vi "Initialize Panel.vi"(7 "Main VI":refnum<vi>, 8 "Error In":errorcluster, 10 "Messages In":refnum<queue>, 11 "State In":T1) -> (0 "Error Out":errorcluster, 2 "Messages Out":refnum<queue>, 3 "State Out":T1)   [LabVIEW 2018, in "Bookmark Manager.lvlib"]
uses:
  Bookmark Manager.lvlib
  Controls/State.ctl
  <vilib>/addons/analyzer/_analyzerctrls.llb/VIAnCtl Analysis App Info.ctl
  Controls/Bookmark.ctl
  Controls/VI Identifier.ctl
  Controls/Bookmarks Groups.ctl
  Controls/Message.ctl
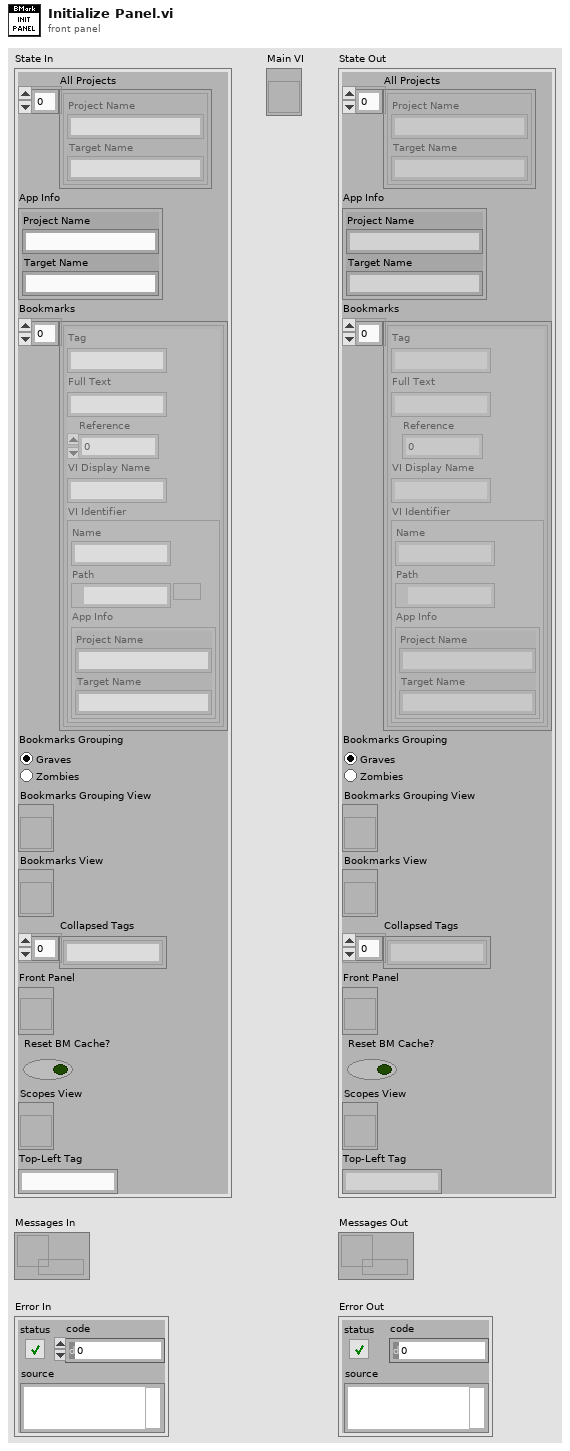
[diagram p1: front panel]
types:
  T1 = typedef "Bookmark Manager.lvlib/State.ctl" = cluster{"All Projects":T2[], "App Info":T2, "Bookmarks":T3[], "Bookmarks Grouping":T5, "Bookmarks Grouping View":refnum<vi>, "Bookmarks View":refnum<vi>, "Collapsed Tags":string[], "Front Panel":refnum<vi>, "Reset BM Cache?":bool, "Scopes View":refnum<vi>, "Top-Left Tag":string}
  T2 = typedef "VIAnCtl Analysis App Info.ctl" = cluster{"Project Name":string, "Target Name":string}
  T3 = typedef "Bookmark Manager.lvlib/Bookmark.ctl" = cluster{"Tag":string, "Full Text":string, "Reference":i32, "VI Display Name":string, "VI Identifier":T4}
  T4 = typedef "Bookmark Manager.lvlib/VI Identifier.ctl" = cluster{"Name":string, "Path":path, "App Info":T2}
  T5 = typedef "Bookmark Manager.lvlib/Bookmarks Groups.ctl" = enum32{"Graves", "Zombies"}
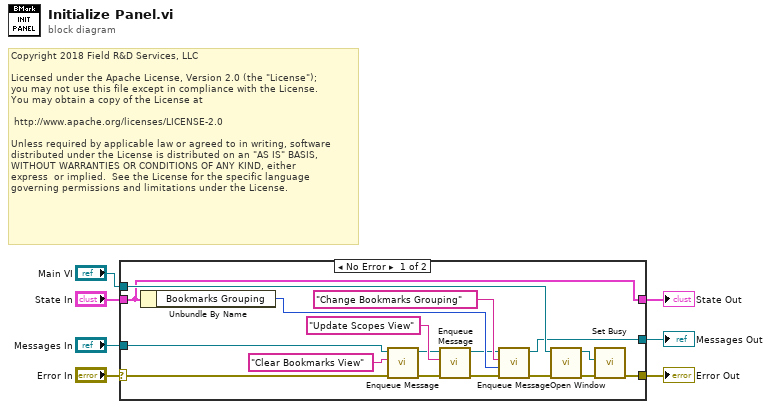
[diagram p0: block diagram]
diagram:
  # "Copyright 2018 Field R&D Services, LLC\n\nLicensed under the Apache License, Version 2.0 (the \"License\");\nyou may not use this file except in compliance with the License.\nYou may obtain a copy of the License at\n\n\thttp://www.apache.org/licenses/LICENSE-2.0\n\nUnless required by applicable law or agreed to in writing, software\ndistributed under the License is distributed on an \"AS IS\" BASIS,\nWITHOUT WARRANTIES OR CONDITIONS OF ANY KIND, either \nexpress  or implied.  See the License for the specific language \ngoverning permissions and limitations under the License."
  n1 = case shown="No Error" "Error In" {
    selector: "Error In" -> [w9 w26]
    tunnel: "State In" -> [w8 w25]
    tunnel: [w15 w26] -> w6
    tunnel: "Main VI" -> [w14 _]
    tunnel: "Messages In" -> [w11 w27]
    tunnel: [w10 w27] -> w3
    tunnel: [w8 w25] -> w1
    frame No Error {
      n2 = Unbundle By Name(w8) -> ("Bookmarks Grouping"=w24:T5)
      n3 = call "Enqueue Message.vi"("Error In"=w9, "Command"="Clear Bookmarks View", "Message Queue In"=w11) -> ("Error Out"=w16:errorcluster, "Message Queue Out"=w19:refnum<queue>)  [unwired: 7 in]
      n4 = call "Enqueue Message.vi"("Error In"=w16, "Command"="Update Scopes View", "Message Queue In"=w19) -> ("Error Out"=w17:errorcluster, "Message Queue Out"=w20:refnum<queue>)  [unwired: 7 in]
      n5 = call "Enqueue Message.vi"("Error In"=w17, "Data"=w24, "Command"="Change Bookmarks Grouping", "Message Queue In"=w20) -> ("Error Out"=w18:errorcluster, "Message Queue Out"=w10:refnum<queue>)  [unwired: 6 in]
      n6 = call "Open Window.vi"("Error In"=w18, "Graveyard Window In"=w14) -> ("Error Out"=w13:errorcluster, "Graveyward Window Out"=w12:refnum<vi>)  [unwired: 7 in, 1 out]
      n7 = call <vilib>:"Set Busy.vi"("error in (no error)"=w13, "VI reference (current VI)"=w12) -> ("error out"=w15:errorcluster)  [unwired: 8 in, 1 out]
    }
    frame Error {
    }
  }
  "Error Out" <- w6
  "Messages Out" <- w3
  "State Out" <- w1
